vi "MerweScSigPts_GetWc.vi"(11 "MerweScaledSigmaPts":T2) -> (3 "Wc":T1)   [LabVIEW 2019, in "Trajectory_Library.lvlib"]
doc: "Creates a new LINEAR SYSTEM data cluster with the specified values. \n\n\nInputs: \n - XXX -- XXX.\n\nOutputs:\n - XXX -- XXX."
uses:
  MERWE_SCALED_SIGMA_PTS.ctl
  <vilib>/Analysis/Matrix/Datatypes/RealMatrix.ctl
  Trajectory_Library.lvlib
  <vilib>/Analysis/Matrix/NI_Matrix.lvlib
panel:
  # "<?, 1>"
  # "<?, 1>"
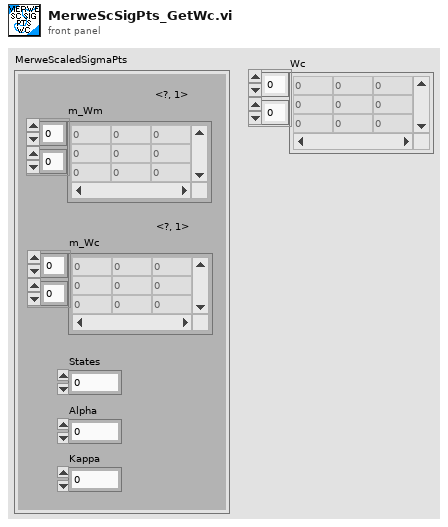
[diagram p1: front panel]
types:
  T1 = typedef "NI_Matrix.lvlib/RealMatrix.ctl" = dbl[][]
  T2 = typedef "Trajectory_Library.lvlib/MERWE_SCALED_SIGMA_PTS.ctl" = cluster{"m_Wm":T1, "States":i32, "Alpha":dbl, "m_Wc":T1, "Kappa":i32}
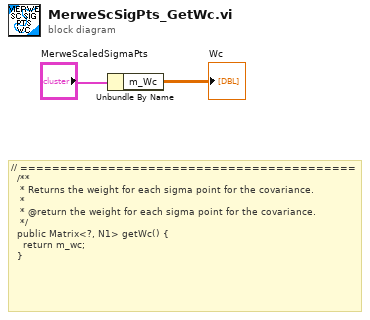
[diagram p0: block diagram]
diagram:
  # "// ==========================================\n  /**\n   * Returns the weight for each sigma point for the covariance.\n   *\n   * @return the weight for each sigma point for the covariance.\n   */\n  public Matrix<?, N1> getWc() {\n    return m_wc;\n  }"
  n1 = Unbundle By Name("MerweScaledSigmaPts") -> ("m_Wc"=→"Wc":T1)
